vi "atributos.vi"(10 "titulo grupo":string) -> (0 "Array 2":dbl[](array[numeric]), 2 "Array":string[](array[string]))   [LabVIEW 2016]
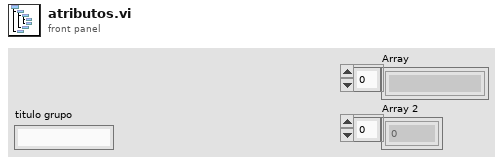
[diagram p1: front panel]
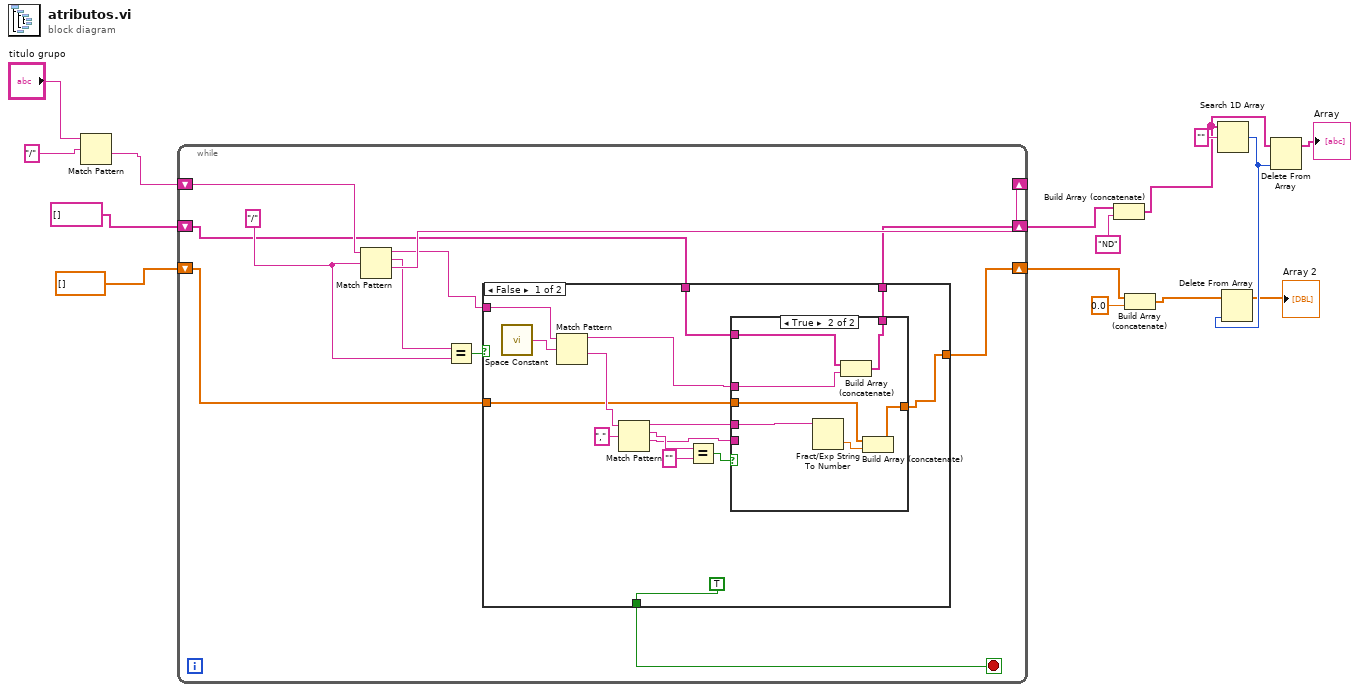
[diagram p0: block diagram]
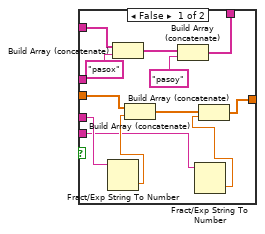
[diagram p2: hidden frame]
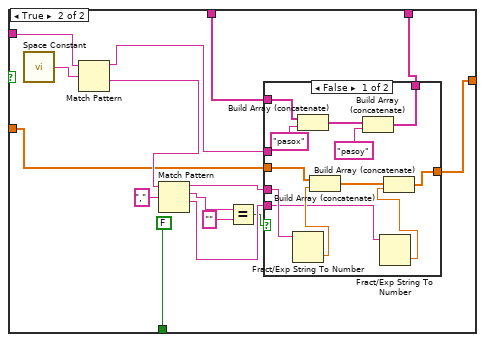
[diagram p3: hidden frame]
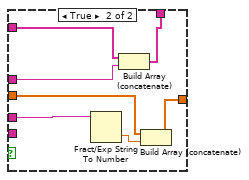
[diagram p4: hidden frame]
diagram:
  n1 = Match Pattern(string="titulo grupo", regular expression="/") -> (after substring=w11:string)  [unwired: 1 in, 3 out]
  n2 = while {
    shift-right: [w16] -> w10
    shift-left: string[] [] -> [w18]
    shift-right: [w17] -> w4
    shift-left: dbl[] [] -> [w19]
    shift-right: [w25] -> _
    shift-left: w11 -> [w26]
    stop <- w21 stop-if-true
    w23 = "/" ("regular expression")
    n3 = Match Pattern(string=w26, regular expression=w23) -> (before substring=w20:string, match substring=w24:string, after substring=w25:string)  [unwired: 1 in, 1 out]
    n4 = Equal?(x=w24, y=w23) -> (x = y?=w22:bool)
    n5 = case shown="False" w22 {
      tunnel: [TRUE FALSE] -> w21
      tunnel: w20 -> [w41 w73]
      tunnel: [w31 w69] -> w17
      tunnel: w19 -> [w30 w61]
      tunnel: [w29 w70] -> w16
      tunnel: w18 -> [w28 w72]
      frame False {
        n6 = call <vilib>:"Space Constant.vi"() -> ("String"=w40:string)
        n7 = Match Pattern(string=w41, regular expression=w40) -> (before substring=w32:string, after substring=w37:string)  [unwired: 1 in, 2 out]
        n8 = Match Pattern(string=w37, regular expression=",") -> (before substring=w35:string, match substring=w34:string, after substring=w27:string)  [unwired: 1 in, 1 out]
        n9 = Equal?(x=w34, y="") -> (x = y?=w36:bool)
        n10 = case shown="True" w36 {
          tunnel: w35 -> [w48 w60]
          tunnel: w32 -> [_ w56]
          tunnel: [w42 w57] -> w31
          tunnel: w30 -> [w47 w59]
          tunnel: [w51 w54] -> w29
          tunnel: w28 -> [w52 w55]
          tunnel: w27 -> [w44 _]
          frame False {
            n11 = Fract/Exp String To Number(string=w48) -> (number=w46:dbl)  [unwired: 3 in, 1 out]
            n12 = Build Array (concatenate)(w52, "pasox") -> (w53:string[])
            n13 = Build Array (concatenate)(w47, w46) -> (w45:dbl[])
            n14 = Build Array (concatenate)(w53, "pasoy") -> (w51:string[])
            n15 = Fract/Exp String To Number(string=w44) -> (number=w43:dbl)  [unwired: 3 in, 1 out]
            n16 = Build Array (concatenate)(w45, w43) -> (w42:dbl[])
          }
          frame True {
            n17 = Fract/Exp String To Number(string=w60) -> (number=w58:dbl)  [unwired: 3 in, 1 out]
            n18 = Build Array (concatenate)(w55, w56) -> (w54:string[])
            n19 = Build Array (concatenate)(w59, w58) -> (w57:dbl[])
          }
        }
      }
      frame True {
        n20 = call <vilib>:"Space Constant.vi"() -> ("String"=w74:string)
        n21 = Match Pattern(string=w73, regular expression=w74) -> (before substring=w71:string, after substring=w65:string)  [unwired: 1 in, 2 out]
        n22 = Match Pattern(string=w65, regular expression=",") -> (before substring=w64:string, match substring=w67:string, after substring=w63:string)  [unwired: 1 in, 1 out]
        n23 = Equal?(x=w67, y="") -> (x = y?=w62:bool)
        n24 = case shown="False" w62 {
          tunnel: w64 -> [w82 w94]
          tunnel: w71 -> [_ w90]
          tunnel: [w76 w91] -> w69
          tunnel: w61 -> [w81 w93]
          tunnel: [w85 w88] -> w70
          tunnel: w72 -> [w86 w89]
          tunnel: w63 -> [w78 _]
          frame False {
            n25 = Fract/Exp String To Number(string=w82) -> (number=w80:dbl)  [unwired: 3 in, 1 out]
            n26 = Build Array (concatenate)(w86, "pasox") -> (w87:string[])
            n27 = Build Array (concatenate)(w81, w80) -> (w79:dbl[])
            n28 = Build Array (concatenate)(w87, "pasoy") -> (w85:string[])
            n29 = Fract/Exp String To Number(string=w78) -> (number=w77:dbl)  [unwired: 3 in, 1 out]
            n30 = Build Array (concatenate)(w79, w77) -> (w76:dbl[])
          }
          frame True {
            n31 = Fract/Exp String To Number(string=w94) -> (number=w92:dbl)  [unwired: 3 in, 1 out]
            n32 = Build Array (concatenate)(w89, w90) -> (w88:string[])
            n33 = Build Array (concatenate)(w93, w92) -> (w91:dbl[])
          }
        }
      }
    }
  }
  n34 = Build Array (concatenate)(w10, "ND") -> (w6:string[])
  n35 = Build Array (concatenate)(w4, 0.0) -> (w1:dbl[])
  n36 = Search 1D Array(1D array=w6, element="") -> (index of element=w3:i32)  [unwired: 1 in]
  n37 = Delete From Array(array=w1, index=w3) -> (array with subset deleted=→"Array 2":dbl[])  [unwired: 1 in, 1 out]
  n38 = Delete From Array(array=w6, index=w3) -> (array with subset deleted=→"Array":string[])  [unwired: 1 in, 1 out]
